vi "FactorPass.vi"(8 "error in (no error)":errorcluster, 9 "OffensivePlay":T1, 10 "Game":refnum<class "Game.lvclass">, 11 "Utilities in":refnum<class "Utilities.lvclass">) -> (0 "error out":errorcluster, 2 "Critério de marcação Normalizado":dbl, 3 "Utilities out":refnum<class "Utilities.lvclass">)   [LabVIEW 2023, in "Utilities.lvclass"]
uses:
  Utilities.lvclass
  Game_class/Game.lvclass
  Team_class/OffensivePlay.ctl
  Robot_class/roles.ctl
  Game_class/Game.lvclass/Game.ctl
  Object_class/Object.lvclass/Object.ctl
  Referee_class/Referee.lvclass/Referee.ctl
  Team_class/Team.lvclass/Team.ctl
  Robot_class/Robot.lvclass/Robot.ctl
  <vilib>/Analysis/_algsub.llb/Real Vector Norm.vi
  Object_class/Read x.vi
  Object_class/Read y.vi
  Robot_class/Read id.vi
  40316e39-9fcb-4662-8d02-ffa9e406c10e.vi
  Game_class/Read BallRef.vi
  Game_class/Read Referee.vi
  Game_class/Read FieldRef.vi
  Game_class/Read EnemyRef.vi
  Game_class/Read Utilities.lvclass.vi
  Game_class/Read OffensiveTeam.vi
  Team_class/Read RobotRef.vi
  Referee_class/Read enemy_goalie_id.vi
  <vilib>/Array/Sort 2D Array - Pop Stack.vi
  <vilib>/Array/Sort 2D Array - Push Stack.vi
  40316e39-9fcb-4662-8d02-ffa9e406c10e.vi/269d4b3b-47f5-49e3-8884-44851e4dd9d5.vi
  40316e39-9fcb-4662-8d02-ffa9e406c10e.vi/6d99389c-673d-4efb-bf33-19b32bcf4cf8.vi
  Ally_class/Ally.lvclass
  C:/Users/roboi/Downloads/VSS_AI-Larc2023/Team_class/Team.lvclass
  Robot_class/Robot.lvclass
  C:/Users/roboi/Downloads/VSS_AI-Larc2023/Object_class/Object.lvclass
  Enemy_class/Enemy.lvclass
  Ball_class/Ball.lvclass
  Referee_class/Referee.lvclass
  Field_class/Field.lvclass
  <vilib>/Analysis/NI_AALPro.lvlib
panel:
  out "t":dbl
  out "id inimigo \nmaior diferença \nde tempo":dbl
  out "Array out":dbl[][](array[numeric])
  out "Dif. tempo\ninimigo bola":dbl
  out "menor dist":dbl
  out "Robô marcado?":bool=TRUE
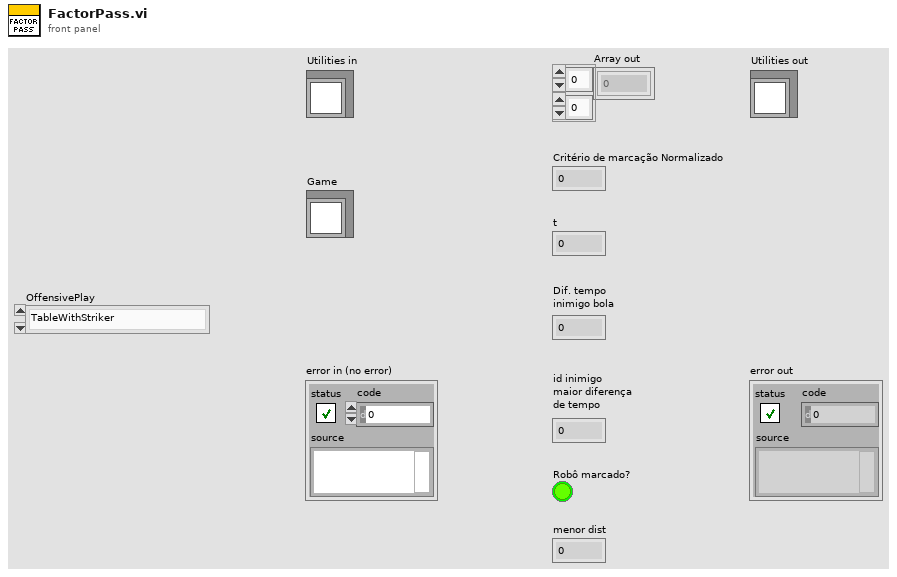
[diagram p1: front panel]
types:
  T1 = typedef "OffensivePlay.ctl" = enum16{"TableWithStriker", "TableWith2ndStrikerPlay", "PrepareDoublePass", "PrepareRollToPass", "SimplePass", "PreparePass", "PassToStriker", "BallOutOfField", "PassTo2ndStriker", "StopOffensive", "Prepare Penalty Enemy", "EnemyPossessionAtEnemyField", "EnemyPossesionAtOurField", "TestPlay", "PreparePenaltyAlly", "KickPenaltyAlly", "PrepareKickoffAlly", "PrepareKickoffEnemy", "IndirectEnemy", "DirectEnemy", "NormalGame", "DirectKick", "Pass", "Halt", "Timeout", "PassPlay", "PenaltyEnemy"}
  T2 = typedef "roles.ctl" = enum16{"BallChallengerAttackerVSS", "NormalAttackerVSS", "AttackerAimGoalVSS", "DefenderAreaVSS", "KeeperVSS", "Tabler", "TableFinalizer", "PrepareRollToPassRoller", "PrepareRollToPassReceiver", "SimplePassRoll", "SimplePassRollReceiver", "PenaltyDefense", "PreparePassReceiver 2", "PreparePassReceiver 1", "PassObserver", "Timeout", "Goto", "ZigZag", "None", "BallOutOfField", "DefenderArea", "Duelist", "AttackerStop", "FollowAttacker", "KeeperRole", "KickPenalty", "AttackerAimGoal", "AttackerBlock", "Marker", "Halt", "Shoot", "PassKicker", "PassReceiver", "TestRole", "PenaltyAttacker"}
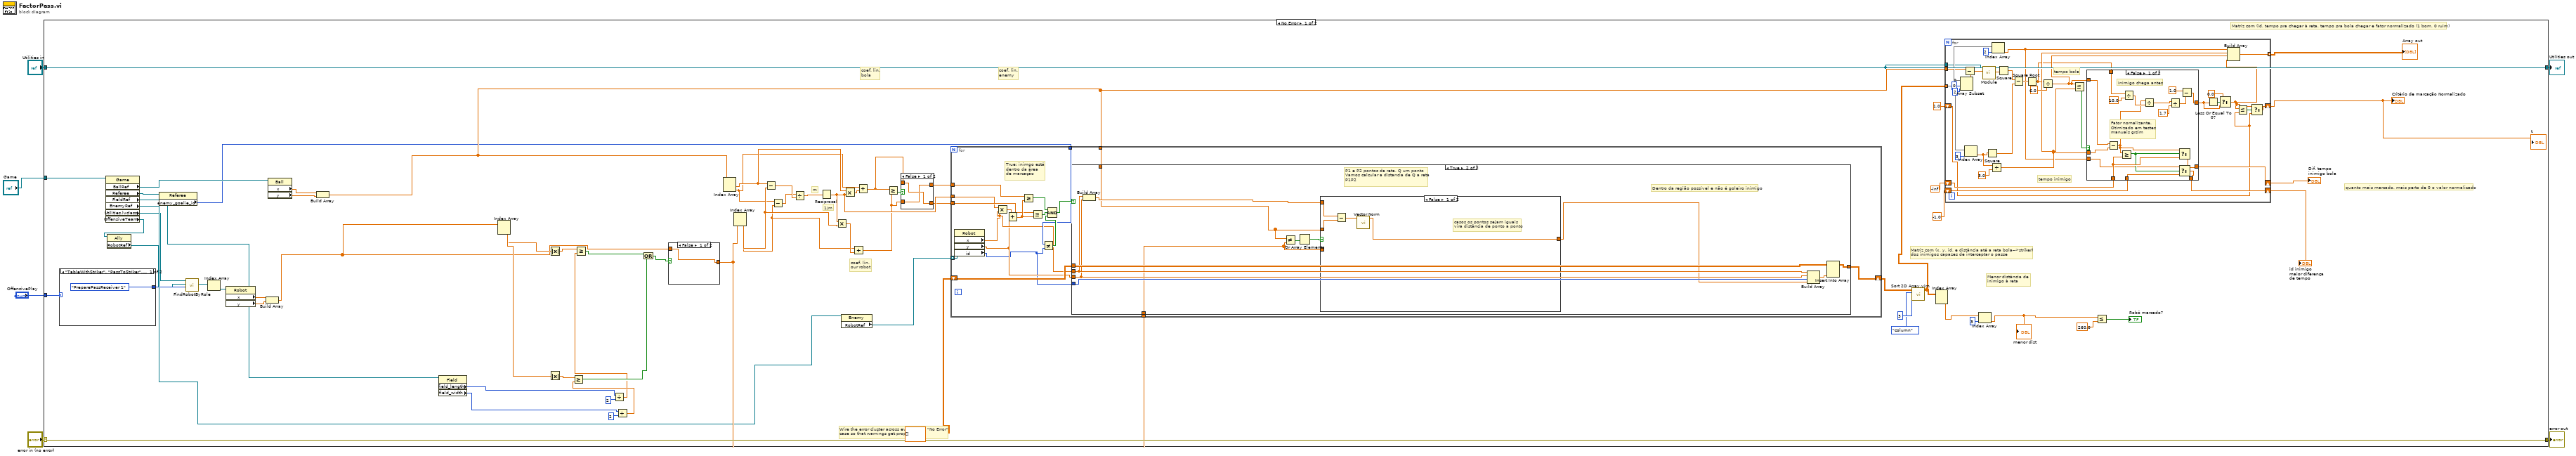
[diagram p0: block diagram]
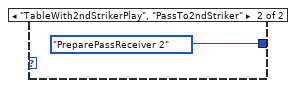
[diagram p2: hidden frame]
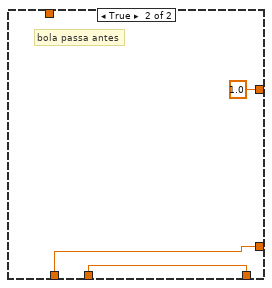
[diagram p3: hidden frame]
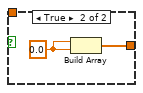
[diagram p4: hidden frame]
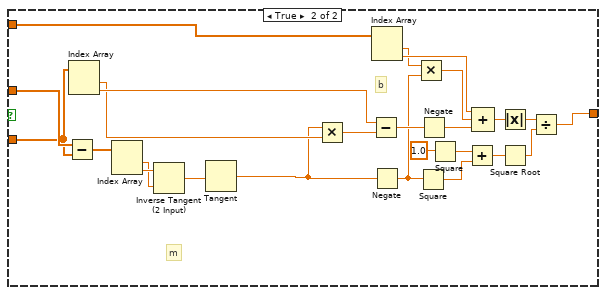
[diagram p7: hidden frame]
diagram:
  n1 = case shown="No Error" "error in (no error)" {
    selector: "error in (no error)" -> [w74 w198]
    tunnel: [w74 w198] -> w5
    tunnel: [w18 w197] -> w3
    tunnel: "Utilities in" -> [w18 w197]
    tunnel: "Game" -> [w17 _]
    tunnel: "OffensivePlay" -> [w16 _]
    frame No Error {
      # "Matriz com (id, tempo pra chegar à reta, tempo pra bola chegar e fator normalizado (1 bom, 0 ruim)"
      # "quanto mais marcado, mais perto de 0 o valor normalizado"
      # "Menor distância de \ninimigo à reta"
      # "Matriz com (x, y, id, e distância até a reta bola-->striker) \ndos inimigos capazes de interceptar o passe"
      # "coef. lin.\nbola"
      # "coef. lin.\nenemy"
      # "coef. lin.\nour robot"
      # "1/m"
      # "m"
      # "Wire the error cluster across even in the \"No Error\"\ncase so that warnings get propagated."
      n2 = case shown="\"TableWithStriker\", \"PassToStriker\", Default" w16 {
        tunnel: [roles."PreparePassReceiver 1" ("role") roles."PreparePassReceiver 2" ("role")] -> w15
        frame "TableWithStriker", "PassToStriker", Default {
        }
        frame "TableWith2ndStrikerPlay", "PassTo2ndStriker" {
        }
      }
      n3 = property class="Game"(reference=w17) -> ("BallRef"=w29:refnum<class "Ball.lvclass">, "Referee"=w25:refnum<class "Referee.lvclass">, "FieldRef"=w23:refnum<class "Field.lvclass">, "EnemyRef"=w20:refnum<class "Enemy.lvclass">, "Utilities.lvclass"=w14:refnum<class "Utilities.lvclass">, "OffensiveTeam"=w8:refnum<class "Ally.lvclass">)  [unwired: 1 in, 2 out]
      n4 = property class="Ally"(reference=w8) -> ("RobotRef"=w7:refnum<class "Robot.lvclass">[])  [unwired: 1 in, 2 out]
      n5 = property class="Referee"(reference=w25) -> ("enemy_goalie_id"=w24:i32)  [unwired: 1 in, 2 out]
      n6 = call "FindRobotByRole.vi"("role"=w15, "RobotRef"=w7, "Utilities in"=w14) -> ("Robots"=w13:refnum<class "Robot.lvclass">[])  [unwired: 6 in, 2 out]
      n7 = Index Array(array=w13) -> (element=w12:refnum<class "Robot.lvclass">)  [unwired: 1 in]
      n8 = property class="Robot"(reference=w12) -> ("x"=w11:dbl, "y"=w10:dbl)  [unwired: 1 in, 2 out]
      n9 = Build Array(w11, w10) -> (w9:dbl[])
      n10 = property class="Ball"(reference=w29) -> ("x"=w28:dbl, "y"=w27:dbl)  [unwired: 1 in, 2 out]
      n11 = Build Array(w28, w27) -> (w26:dbl[])
      n12 = property class="Field"(reference=w23) -> ("field_length"=w22:i32, "field_width"=w21:i32)  [unwired: 1 in, 2 out]
      n13 = Index Array(array=w9) -> (element #1=w69:dbl, element #2=w70:dbl)  [unwired: 2 in]
      n14 = Absolute Value(x=w69) -> (abs(x)=w49:dbl)
      n15 = Absolute Value(x=w70) -> (abs(x)=w51:dbl)
      n16 = Divide(x=w22, y=2) -> (x/y=w50:dbl)
      n17 = Greater Or Equal?(x=w49, y=w50) -> (x >= y?=w53:bool)
      n18 = Divide(x=w21, y=u32 2) -> (x/y=w52:dbl)
      n19 = Greater Or Equal?(x=w51, y=w52) -> (x >= y?=w54:bool)
      n20 = Or(x=w53, y=w54) -> (x .or. y?=w55:bool)
      n21 = case shown="False" w55 {
        tunnel: [w130 w131] -> w56
        tunnel: w9 -> [w130 _]
        frame False {
        }
        frame True {
          w132 = 0.0
          n22 = Build Array(w132, w132) -> (w131:dbl[])
        }
      }
      n23 = Index Array(array=w26) -> (element #1=w66:dbl, element #2=w31:dbl)  [unwired: 2 in]
      n24 = Index Array(array=w56) -> (element #1=w65:dbl, element #2=w32:dbl)  [unwired: 2 in]
      n25 = Subtract(x=w66, y=w65) -> (x-y=w34:dbl)
      n26 = Subtract(x=w31, y=w32) -> (x-y=w33:dbl)
      n27 = Divide(x=w33, y=w34) -> (x/y=w30:dbl)
      n28 = Reciprocal(x=w30) -> (1/x=w68:dbl)
      n29 = Multiply(x=w68, y=w65) -> (x*y=w64:dbl)
      n30 = property class="Enemy"(reference=w20) -> ("RobotRef"=w19:refnum<class "Robot.lvclass">[])  [unwired: 1 in, 2 out]
      n31 = Multiply(x=w66, y=w68) -> (x*y=w67:dbl)
      n32 = Add(x=w32, y=w64) -> (x+y=w37:dbl)
      n33 = Add(x=w31, y=w67) -> (x+y=w36:dbl)
      n34 = Greater Or Equal?(x=w36, y=w37) -> (x >= y?=w35:bool)
      n35 = case shown="False" w35 {
        tunnel: [w134 w136] -> w38
        tunnel: w36 -> [w133 w136]
        tunnel: [w133 w135] -> w39
        tunnel: w37 -> [w134 w135]
        frame False {
        }
        frame True {
        }
      }
      n36 = for {
        tunnel: w68 -> [w144]
        shift-right: [w153] -> w42
        shift-left: dbl[][] [] -> [w154]
        tunnel: w38 -> [w148]
        tunnel: w39 -> [w147]
        tunnel: w26 -> [w146]
        tunnel: w56 -> [w145]
        tunnel: w24 -> [w141]
        tunnel: w19 -> [w140] mode=indexing
        # "True: inimgo está \ndentro da área\nde marcação"
        n37 = property class="Robot"(reference=w140) -> ("x"=w139:dbl, "y"=w138:dbl, "id"=w137:i32)  [unwired: 1 in, 2 out]
        n38 = Multiply(x=w144, y=w139) -> (x*y=w143:dbl)
        n39 = Add(x=w143, y=w138) -> (x+y=w152:dbl)
        n40 = Greater Or Equal?(x=w148, y=w152) -> (x >= y?=w150:bool)
        n41 = Less Or Equal?(x=w147, y=w152) -> (x <= y?=w151:bool)
        n42 = Not Equal?(x=w141, y=w137) -> (x != y?=w142:bool)
        n43 = Compound Arithmetic op=AND(w150, w151, w142) -> (w149:bool)
        n44 = case shown="True" w149 {
          tunnel: w154 -> [w155 w167]
          tunnel: [w155 w166] -> w153
          tunnel: w139 -> [_ w163]
          tunnel: w138 -> [_ w162]
          tunnel: w137 -> [_ w165]
          tunnel: w146 -> [_ w158]
          tunnel: w145 -> [_ w157]
          frame False {
            # "Fora da região possível ou é goleiro inimigo"
          }
          frame True {
            # "P1 e P2 pontos da reta, Q um ponto\nVamos calcular a distancia de Q a reta \nP1P2"
            # "Dentro da região possível e não é goleiro inimigo"
            n45 = Build Array(w163, w162) -> (w159:dbl[])
            n46 = Not Equal?(x=w158, y=w157) -> (x != y?=w161:bool[])
            n47 = Or Array Elements(Boolean array=w161) -> (logical OR=w160:bool)
            n48 = case shown="False" w160 {
              tunnel: w158 -> [w170 w196]
              tunnel: w157 -> [_ w192]
              tunnel: w159 -> [w171 w188]
              tunnel: [w168 w174] -> w156
              frame False {
                # "casos os pontos sejam iguais\nvira distância de ponto a ponto"
                n49 = Subtract(x=w171, y=w170) -> (x-y=w169:dbl[])
                n50 = call-poly <vilib>:"Vector Norm.vi"("Input Vector"=w169) -> ("norm"=w168:dbl)  [unwired: 9 in, 1 out]
              }
              frame True {
                # "b"
                # "m"
                n51 = Subtract(x=w196, y=w192) -> (x-y=w195:dbl[])
                n52 = Index Array(array=w192) -> (element #1=w190:dbl, element #2=w191:dbl)  [unwired: 2 in]
                n53 = Index Array(array=w195) -> (element #1=w193:dbl, element #2=w194:dbl)  [unwired: 2 in]
                n54 = Inverse Tangent (2 Input)(1:w193, 2:w194) -> (0:w173:dbl)
                n55 = Tangent(1:w173) -> (0:w172:dbl)
                n56 = Multiply(x=w172, y=w190) -> (x*y=w189:dbl)
                n57 = Subtract(x=w191, y=w189) -> (x-y=w184:dbl)
                n58 = Index Array(array=w188) -> (element #1=w186:dbl, element #2=w187:dbl)  [unwired: 2 in]
                n59 = Negate(x=w172) -> (-x=w180:dbl)
                n60 = Multiply(x=w186, y=w180) -> (x*y=w185:dbl)
                n61 = Square(x=w180) -> (x^2=w178:dbl)
                n62 = Negate(x=w184) -> (-x=w183:dbl)
                n63 = Square(x=1.0) -> (x^2=w179:dbl)
                n64 = Add(x=w179, y=w178) -> (x+y=w177:dbl)
                n65 = Compound Arithmetic op=ADD(w187, w185, w183) -> (w182:dbl)
                n66 = Absolute Value(x=w182) -> (abs(x)=w176:dbl)
                n67 = Square Root(x=w177) -> (sqrt(x)=w175:dbl)
                n68 = Divide(x=w176, y=w175) -> (x/y=w174:dbl)
              }
            }
            n69 = Build Array(w163, w162, w165, w156) -> (w164:dbl[])
            n70 = Insert Into Array(array=w167, new element=w164) -> (w166:dbl[][])  [unwired: 2 in]
          }
        }
      }
      n71 = call "Sort 2D Array.vim"("index"=3, "dimension to index (column)"=enum16{"column", "row"}."column", "2D array"=w42) -> ("sorted 2D array"=w59:dbl[][])  [unwired: 7 in, 1 out]
      n72 = Index Array(array=w59) -> (element=w58:dbl[])  [unwired: 2 in]
      n73 = for {
        tunnel: w26 -> [w80]
        tunnel: w59 -> [w94] mode=indexing
        shift-right: [w90] -> w71
        shift-left: -inf -> [w99]
        tunnel: [w98] -> w61 mode=indexing
        shift-right: [w93] -> w63
        shift-left: -1.0 ("Numeric") -> [w91]
        shift-right: [w85] -> w72
        shift-left: 1.0 ("t") -> [w83]
        tunnel: w18 -> [w78]
        # "tempo inimigo"
        # "tempo bola"
        n74 = Array Subset(array=w94, index=0, length=2) -> (w81:dbl[])
        n75 = Subtract(x=w80, y=w81) -> (x-y=w79:dbl[])
        n76 = Index Array(array=w94, index=3) -> (element=w102:dbl)
        n77 = call-dynamic "Module.vi"("2D vector"=w79, "Utilities in"=w78) -> ("Modulo"=w77:dbl)  [unwired: 7 in, 2 out]
        n78 = Square(x=w102) -> (x^2=w105:dbl)
        n79 = Divide(x=w102, y=3.0) -> (x/y=w96:dbl)
        n80 = Index Array(array=w94, index=2) -> (element=w92:dbl)
        n81 = Square(x=w77) -> (x^2=w106:dbl)
        n82 = Subtract(x=w106, y=w105) -> (x-y=w104:dbl)
        n83 = Square Root(x=w104) -> (sqrt(x)=w89:dbl)
        n84 = Divide(x=w89, y=6.0) -> (x/y=w97:dbl)
        n85 = Less Or Equal?(x=w97, y=w96) -> (x <= y?=w100:bool)
        n86 = case shown="False" w100 {
          tunnel: w96 -> [w124 _]
          tunnel: w97 -> [w125 _]
          tunnel: [w116 w129] -> w90
          tunnel: w99 -> [w126 w129]
          tunnel: [w122 w128] -> w93
          tunnel: w92 -> [w121 _]
          tunnel: w91 -> [w120 w128]
          tunnel: w89 -> [w119 _]
          tunnel: [w111 1.0] -> w87
          frame False {
            # "Fator nomalizante.\nOtimizado em testes\nmanuais grsim"
            # "inimigo chega antes"
            n87 = Subtract(x=w125, y=w124) -> (x-y=w110:dbl)
            n88 = Greater Or Equal?(x=w110, y=w126) -> (x >= y?=w123:bool)
            n89 = Divide(x=w119, y=10.0) -> (x/y=w117:dbl)
            n90 = Divide(x=w110, y=w117) -> (x/y=w115:dbl)
            n91 = Divide(x=w115, y=1.7) -> (x/y=w112:dbl)
            n92 = Select(t=w110, s=w123, f=w126) -> (s? t:f=w116:dbl)
            n93 = Select(t=w121, s=w123, f=w120) -> (s? t:f=w122:dbl)
            n94 = Subtract(x=1.0, y=w112) -> (x-y=w111:dbl)
          }
          frame True {
            # "bola passa antes"
          }
        }
        n95 = Less Or Equal To 0?(x=w87) -> (x <= 0?=w88:bool)
        n96 = Select(t=0.0, s=w88, f=w87) -> (s? t:f=w84:dbl)
        n97 = Build Array(w92, w96, w97, w84) -> (w98:dbl[])
        n98 = Less Or Equal?(x=w84, y=w83) -> (x <= y?=w82:bool)
        n99 = Select(t=w84, s=w82, f=w83) -> (s? t:f=w85:dbl)
      }
      "Dif. tempo\ninimigo bola" <- w71
      "Array out" <- w61
      "id inimigo \nmaior diferença \nde tempo" <- w63
      "Critério de marcação Normalizado" <- w72
      "t" <- w72
      n100 = Index Array(array=w58, index=3) -> (element=w57:dbl)
      "menor dist" <- w57
      n101 = Less Or Equal?(x=w57, y=260.0) -> (x <= y?=→"Robô marcado?":bool)
    }
    frame Error {
    }
  }
  "error out" <- w5
  "Utilities out" <- w3
